vi "8-11-1 생산 소비 이벤트.vi"() -> ()   [LabVIEW 2019]
doc: "이 템플릿을 사용하여 마스터/슬레이브 디자인 패턴을 생성합니다. 마스터 루프는 항상 실행됩니다. 이것은 코드를 실행하기 위해서 하나 이상의 슬래이브 루프에 알립니다. 슬레이브 루프는 이것이 완료될 때까지 계속적으로 실행하고, 다른 알림이 있을 때까지 기다립니다. 이에 비해 생산/소비 패턴에서는 소비 루프의 큐에 데이터가 존재할 때만 소비 루프가 실행됩니다."
panel:
  in  "데이터 전달":bool caption="정지"
  out "수신 데이터":cluster{"이름":string, "토익 점수":dbl}
  in  "송신 데이터":cluster{"이름":string, "토익 점수":dbl}={"이름"="홍길동 ", "토익 점수"=550.0}
  out "소비 루프 반복 횟수":i32
  out "생산 루프 반복 횟수":i32
  in  "stop":bool caption="정지"
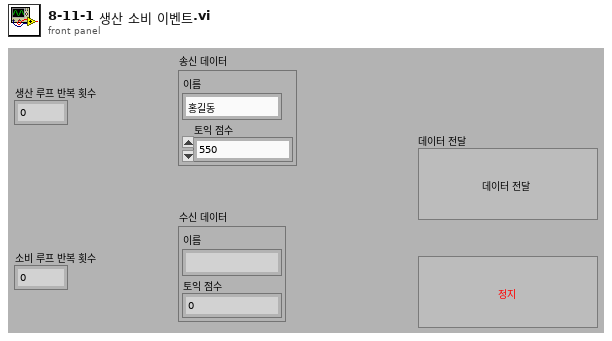
[diagram p1: front panel]
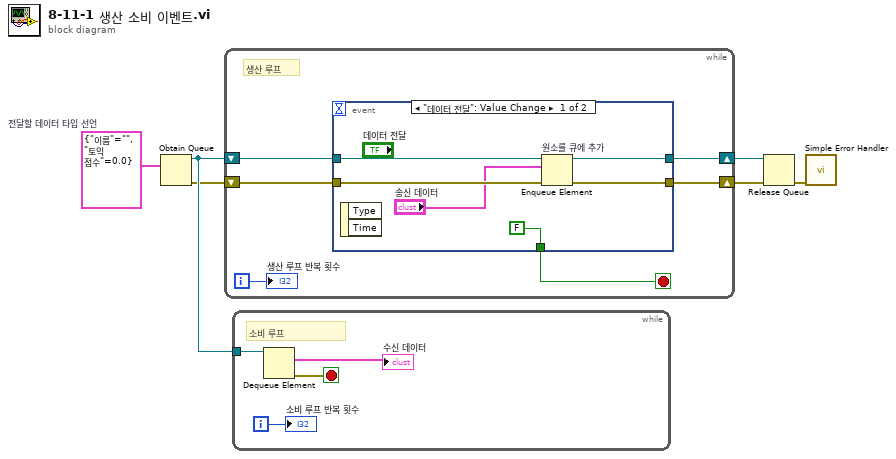
[diagram p0: block diagram]
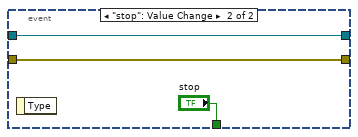
[diagram p2: hidden frame]
diagram:
  w1 = cluster{"이름":string, "토익 점수":dbl} {"이름"="", "토익 점수"=0.0}  # 전달할 데이터 타입 선언
  n1 = Obtain Queue(element data type=w1) -> (queue out=w6:refnum<queue>, error out=w5:errorcluster)  [unwired: 4 in, 1 out]
  n2 = while {
    shift-right: [w11] -> w4
    shift-left: w5 -> [w10]
    shift-right: [w9] -> w3
    shift-left: w6 -> [w12]
    i -> [w8]
    stop <- w7 stop-if-true
    # "생산 루프"
    n3 = event shown="[0] \"데이터 전달\": Value Change" {
      selector: _ -> [_ _]
      dyn-events: _ -> [_ _]
      timeout: _ -> [_ _]
      tunnel: w12 -> [w18 w21]
      tunnel: [w17 w20] -> w11
      tunnel: w10 -> [w16 w20]
      tunnel: [w15 w21] -> w9
      tunnel: [FALSE ("stop") "stop"] -> w7
      event "데이터 전달": Value Change {
        n4 = event-data() -> ()  [unwired: 1 in, 2 out]
        n5 = Enqueue Element "원소를 큐에 추가"(queue=w18, element="송신 데이터", error in (no error)=w16) -> (queue out=w15:refnum<queue>, error out=w17:errorcluster)  [unwired: 1 in, 1 out]
      }
      event "stop": Value Change {
        n6 = event-data() -> ()  [unwired: 1 in, 1 out]
      }
    }
    "생산 루프 반복 횟수" <- w8
  }
  n7 = while {
    tunnel: w6 -> [w25]
    i -> [w23]
    stop <- w24 stop-if-true
    # "소비 루프"
    n8 = Dequeue Element(queue=w25) -> (element=→"수신 데이터":cluster{"이름":string, "토익 점수":dbl}, error out=w24:errorcluster)  [unwired: 2 in, 2 out]
    "소비 루프 반복 횟수" <- w23
  }
  n9 = Release Queue(queue=w3, error in (no error)=w4) -> (error out=w2:errorcluster)  [unwired: 1 in, 2 out]
  n10 = call <vilib>:"Simple Error Handler.vi"("error in (no error)"=w2) -> ()  [unwired: 4 in, 5 out]
